vi "Convert Pulses to Flow Rate.vi"(8 "Time Range":dbl=60.0, 9 "K":dbl, 11 "Pulses / sec":u32) -> (3 "Flow Rate":dbl)   [LabVIEW 2017]
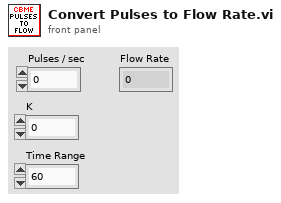
[diagram p1: front panel]
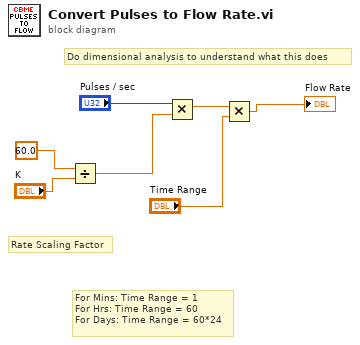
[diagram p0: block diagram]
diagram:
  # "Do dimensional analysis to understand what this does"
  # "For Mins: Time Range = 1\nFor Hrs: Time Range = 60\nFor Days: Time Range = 60*24"
  # "Rate Scaling Factor"
  n1 = Divide(x=60.0, y="K") -> (x/y=w6:dbl)
  n2 = Multiply(x="Pulses / sec", y=w6) -> (x*y=w4:dbl)
  n3 = Multiply(x=w4, y="Time Range") -> (x*y=→"Flow Rate":dbl)
